vi "CalculateOffsetMRay.vi"(9 "AR2":dbl, 11 "AR1":dbl) -> (2 "Offset":dbl)   [LabVIEW 2011]
panel:
  in  "x":dbl=0.33
  # "0.33 Last Offset"
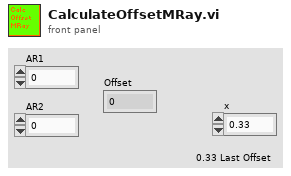
[diagram p1: front panel]
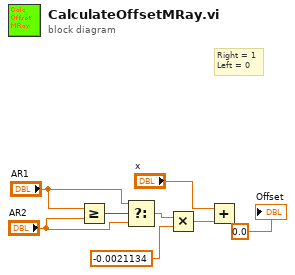
[diagram p0: block diagram]
diagram:
  # "Right = 1\nLeft = 0"
  n1 = Greater Or Equal?(x="AR1", y="AR2") -> (x >= y?=w8:bool)
  n2 = Select(t="AR1", s=w8, f="AR2") -> (s? t:f=w5:dbl)
  n3 = Multiply(x=w5, y=-0.0021134) -> (x*y=w3:dbl)
  n4 = Add(x="x", y=w3) -> ()  [unwired: 1 out]
  "Offset" <- 0.0 ("Offset")
